vi "QueryGrating.vi"(8 "error in (no error)":errorcluster, 11 "HRS_Spectrometer in":refnum<class "HRS_Spectrometer.lvclass">) -> (0 "error out":errorcluster, 3 "HRS_Spectrometer out":refnum<class "HRS_Spectrometer.lvclass">)   [LabVIEW 2023, in "HRS_Spectrometer.lvlib" / "HRS_Spectrometer.lvclass"]
uses:
  HRS_Spectrometer.lvclass
  HRS_Spectrometer.lvclass/HRS_Spectrometer.ctl
  <vilib>/addons/Tools/Unicode/UTF8 Tools.lvlib
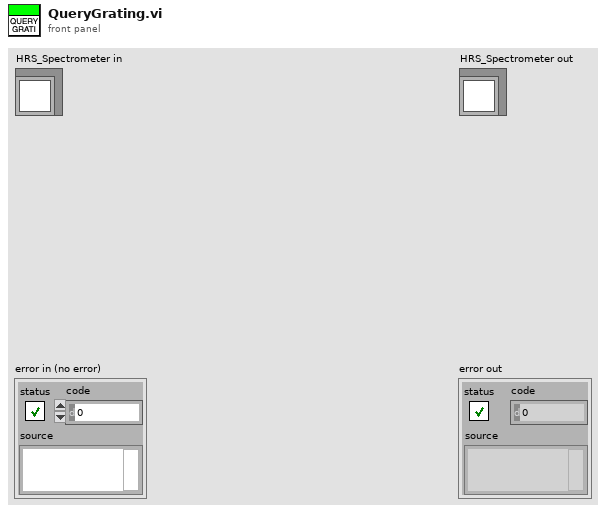
[diagram p1: front panel]
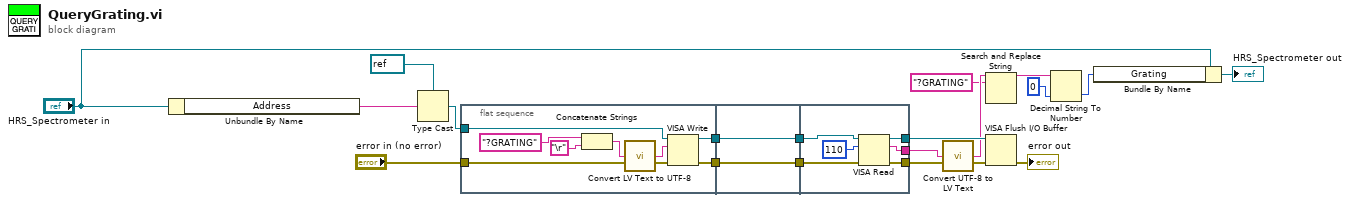
[diagram p0: block diagram]
diagram:
  n1 = Unbundle By Name("HRS_Spectrometer in") -> ("Address"=w14:string)
  n2 = Type Cast(type=refnum<visa-resource-name> refnum ("VISA resource name out"), x=w14) -> (*(type *) &x=w10:refnum<visa-resource-name>)
  n3 = flat-sequence {
    tunnel: [w29] -> w20
    tunnel: [w28] -> w19
    tunnel: w10 -> [w27]
    tunnel: "error in (no error)" -> [w24]
    tunnel: w20 -> [w31]
    tunnel: w19 -> [w30]
    tunnel: [w31] -> w8
    tunnel: [w30] -> w7
    tunnel: [w37] -> w12
    tunnel: [w36] -> w11
    tunnel: [w35] -> w6
    tunnel: w8 -> [w33]
    tunnel: w7 -> [w32]
    frame #0 {
      n4 = Concatenate Strings("?GRATING" ("write buffer"), "\r") -> (w21:string)
      n5 = call <vilib>:"Convert LV Text to UTF-8.vi"("LV Text"=w21, "error in"=w24) -> ("UTF-8 Text"=w26:string, "error out"=w25:errorcluster)  [unwired: 12 in]
      n6 = VISA Write(VISA resource name=w27, write buffer=w26, error in (no error)=w25) -> (VISA resource name out=w29:refnum<visa-resource-name>, error out=w28:errorcluster)  [unwired: 1 out]
    }
    frame #1 {
    }
    frame #2 {
      n7 = VISA Read(VISA resource name=w33, byte count=u32 110, error in (no error)=w32) -> (VISA resource name out=w35:refnum<visa-resource-name>, read buffer=w37:string, error out=w36:errorcluster)  [unwired: 1 out]
    }
  }
  n8 = call <vilib>:"Convert UTF-8 to LV Text.vi"("UTF-8 Text"=w12, "error in"=w11) -> ("LV Text"=w3:string, "error out"=w5:errorcluster)  [unwired: 12 in]
  n9 = Search and Replace String(input string=w3, search string="?GRATING") -> (result string=w1:string)  [unwired: 6 in, 3 out]
  n10 = VISA Flush I/O Buffer(VISA resource name=w6, error in (no error)=w5) -> (error out=→"error out":errorcluster)  [unwired: 1 in, 1 out]
  n11 = Decimal String To Number(string=w1, default (0L)=0 ("default (0 I32)")) -> (number=w16:i32)  [unwired: 1 in, 1 out]
  n12 = Bundle By Name(cluster="HRS_Spectrometer in", "Grating"=w16) -> (→"HRS_Spectrometer out":refnum<class "HRS_Spectrometer.lvclass">)
